vi "CNR compute LAR weights.vi"(11 "residuals":dbl[](array[numeric])) -> (3 "LAR weights":dbl[](array[numeric]))   [LabVIEW 2020, in "NI_Gmath.lvlib"]
uses:
  NI_Gmath.lvlib
panel:
  out "error out":errorcluster
  in  "error in (no error)":errorcluster
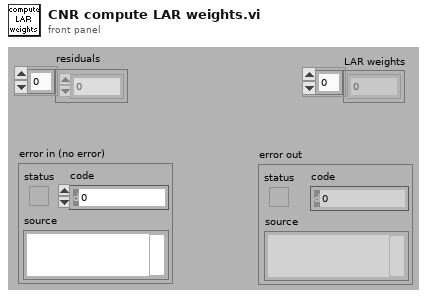
[diagram p1: front panel]
types:
  T1 = enum16{"arithmetic", "geometric", "harmonic", "trimmed", "median"}
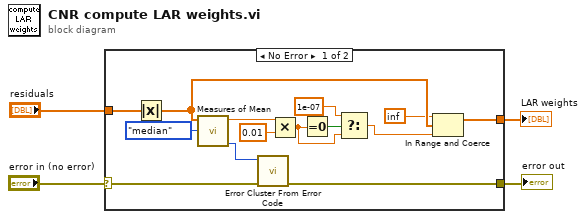
[diagram p0: block diagram]
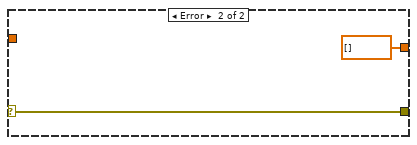
[diagram p2: hidden frame]
diagram:
  n1 = case shown="No Error" "error in (no error)" {
    selector: "error in (no error)" -> [w6 w20]
    tunnel: "residuals" -> [w18 _]
    tunnel: [w8 dbl[] []] -> w3
    tunnel: [w5 w20] -> w1
    frame No Error {
      n2 = Absolute Value(x=w18) -> (abs(x)=w10:dbl[])
      n3 = call "Measures of Mean.vi"("type"=T1."median", "x array"=w10) -> ("error"=w7:i32, "mean value"=w16:dbl)  [unwired: 8 in]
      n4 = call "Error Cluster From Error Code.vi"("error in (no error)"=w6, "error code (0)"=w7) -> ("error out"=w5:errorcluster)  [unwired: 7 in]
      n5 = Multiply(x=w16, y=0.01) -> (x*y=w13:dbl)
      n6 = Equal To 0?(x=w13) -> (x = 0?=w14:bool)
      n7 = Select(t=1e-07, s=w14, f=w13) -> (s? t:f=w11:dbl)
      n8 = In Range and Coerce(upper limit=inf, x=w10, lower limit=w11) -> (coerced(x)=w8:dbl[])  [unwired: 1 out]
    }
    frame Error {
    }
  }
  "LAR weights" <- w3
  "error out" <- w1
